vi "Build Message Parameters.vi"(8 "error in (no error)":errorcluster, 11 "Message XML Node":refnum<k20>) -> (0 "error out":errorcluster, 3 "Parameters":T1[](array[typedef]) {"Base Word" format="%04d"; "Address" format="%04x"; "Mask" format="%04x"; "Value" format="%016x"})   [LabVIEW 2016]
doc: "Retrieves all the XML information for defining parameters/channels that are encoded in/decoded from the Message data words. Each parameter/channel should have a unique name."
uses:
  <vilib>/xml/NI_XML.lvlib
  1553 SubComponent/TypeDefs/Scaling Information.ctl
  1553 SubComponent/1553 SubComponent.lvclass
  1553 SubComponent/TypeDefs/Parameter Table Data.ctl
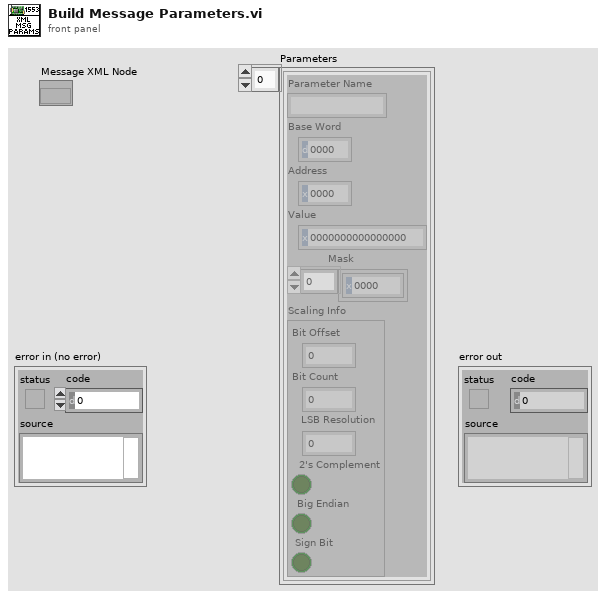
[diagram p1: front panel]
types:
  T1 = typedef "BCI-1553 API.lvlib/1553 SubComponent.lvclass/Parameter Table Data.ctl" = cluster{"Parameter Name":string, "Base Word":u16, "Address":u16, "Value":u64, "Mask":u16[], "Scaling Info":T2}
  T2 = typedef "BCI-1553 API.lvlib/1553 SubComponent.lvclass/Scaling Information.ctl" = cluster{"Bit Offset":i32, "Bit Count":i32, "LSB Resolution":dbl, "2's Complement":bool, "Big Endian":bool, "Sign Bit":bool}
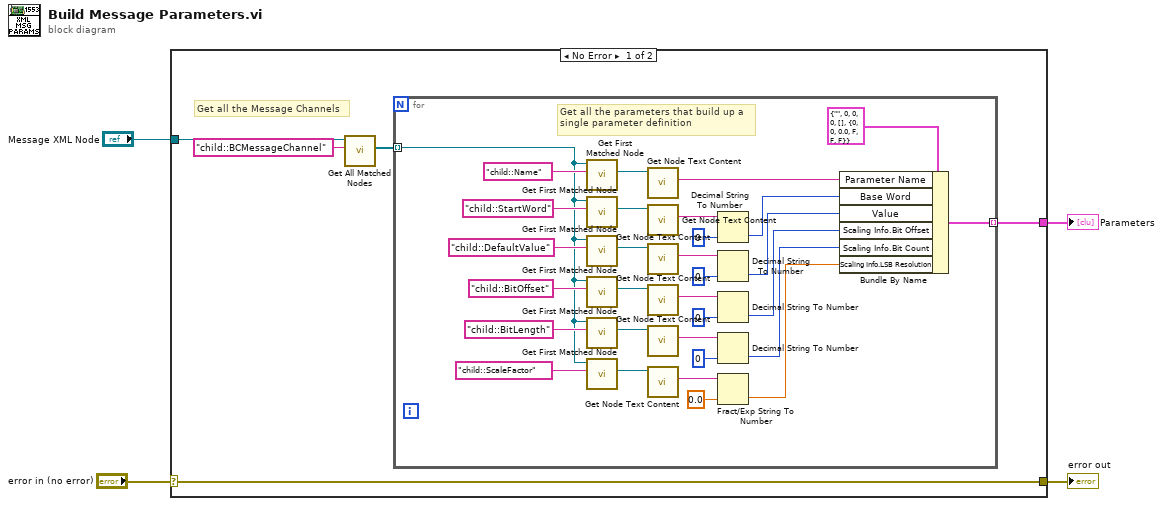
[diagram p0: block diagram]
diagram:
  n1 = case shown="No Error" "error in (no error)" {
    selector: "error in (no error)" -> [w9 w41]
    tunnel: [w9 w41] -> w3
    tunnel: "Message XML Node" -> [w8 _]
    tunnel: [w6 _] -> w1
    frame No Error {
      # "Get all the Message Channels"
      n2 = call <vilib>:"Get All Matched Nodes.vi"("XPath expression"="child::BCMessageChannel", "node in"=w8) -> ("node result array"=w5:refnum<k20>[])  [unwired: 7 in, 2 out]
      n3 = for {
        tunnel: w5 -> [w14] mode=indexing
        tunnel: [w39] -> w6 mode=indexing
        # "Get all the parameters that build up a\nsingle parameter definition"
        n4 = call <vilib>:"Get First Matched Node.vi"("XPath expression"="child::Name", "node in"=w14) -> ("node result"=w37:refnum<k20>)  [unwired: 7 in, 2 out]
        n5 = call <vilib>:"Get First Matched Node.vi"("XPath expression"="child::StartWord", "node in"=w14) -> ("node result"=w35:refnum<k20>)  [unwired: 7 in, 2 out]
        n6 = call <vilib>:"Get First Matched Node.vi"("XPath expression"="child::DefaultValue", "node in"=w14) -> ("node result"=w28:refnum<k20>)  [unwired: 7 in, 2 out]
        n7 = call <vilib>:"Get First Matched Node.vi"("XPath expression"="child::BitOffset", "node in"=w14) -> ("node result"=w25:refnum<k20>)  [unwired: 7 in, 2 out]
        n8 = call <vilib>:"Get First Matched Node.vi"("XPath expression"="child::BitLength", "node in"=w14) -> ("node result"=w17:refnum<k20>)  [unwired: 7 in, 2 out]
        n9 = call <vilib>:"Get First Matched Node.vi"("XPath expression"="child::ScaleFactor", "node in"=w14) -> ("node result"=w15:refnum<k20>)  [unwired: 7 in, 2 out]
        n10 = call <vilib>:"Get Node Text Content.vi"("node in"=w37) -> ("node text"=w36:string)  [unwired: 8 in, 2 out]
        n11 = call <vilib>:"Get Node Text Content.vi"("node in"=w35) -> ("node text"=w33:string)  [unwired: 8 in, 2 out]
        n12 = call <vilib>:"Get Node Text Content.vi"("node in"=w28) -> ("node text"=w30:string)  [unwired: 8 in, 2 out]
        n13 = call <vilib>:"Get Node Text Content.vi"("node in"=w25) -> ("node text"=w23:string)  [unwired: 8 in, 2 out]
        n14 = call <vilib>:"Get Node Text Content.vi"("node in"=w17) -> ("node text"=w19:string)  [unwired: 8 in, 2 out]
        n15 = call <vilib>:"Get Node Text Content.vi"("node in"=w15) -> ("node text"=w13:string)  [unwired: 8 in, 2 out]
        n16 = Decimal String To Number(string=w33, default (0L)=u16 0 ("Base Word")) -> (number=w31:u16)  [unwired: 1 in, 1 out]
        n17 = Decimal String To Number(string=w30, default (0L)=u64 0 ("Value")) -> (number=w26:u64)  [unwired: 1 in, 1 out]
        n18 = Decimal String To Number(string=w23, default (0L)=0 ("default (0 I32)")) -> (number=w22:i32)  [unwired: 1 in, 1 out]
        n19 = Decimal String To Number(string=w19, default (0L)=0 ("default (0 I32)")) -> (number=w16:i32)  [unwired: 1 in, 1 out]
        n20 = Fract/Exp String To Number(string=w13, default (0 dbl)=0.0 ("default (0 DBL)")) -> (number=w12:dbl)  [unwired: 2 in, 1 out]
        n21 = Bundle By Name(cluster=T1 {"Parameter Name"="", "Base Word"=0, "Address"=0, "Value"=0, "Mask"=[], "Scaling Info"={"Bit Offset"=0, "Bit Count"=0, "LSB Resolution"=0.0, "2's Complement"=FALSE, "Big Endian"=FALSE, "Sign Bit"=FALSE}} ("Parameter Table Data"), "Parameter Name"=w36, "Base Word"=w31, "Value"=w26, "Scaling Info.Bit Offset"=w22, "Scaling Info.Bit Count"=w16, "Scaling Info.LSB Resolution"=w12) -> (w39:T1)
      }
    }
    frame Error {
    }
  }
  "error out" <- w3
  "Parameters" <- w1
